vi "通道配置模块.vi"() -> (1 "返回":bool)   [LabVIEW 2010]
uses:
  全局量/试验配置信息.vi
  全局量/全局_配置.vi
  <vilib>/Utility/config.llb/Write Key (String).vi
  <vilib>/Utility/config.llb/Write Key (I32).vi
  <vilib>/Utility/config.llb/NI_LVConfig.lvlib
panel:
  out "temp":string[](array[string])
  in  "Row":i32
  in  "模拟量误差":dbl format="%.4f"
  out "配置文件目录":path
  out "配置文件路径":path
  out "配置文件目录 2":path
  out "配置文件路径 2":path
  in  "选项卡控件 2":enum32{"选项卡 1", "选项卡 2"}(tab)
  in  "模拟量误差百分比":dbl
  in  "数字量输出路数":u32=1 max=76
  in  "数字量输入路数":u32 max=80
  in  "DSP输入路数":u32 max=16
  in  "DSP输入幅值":enum32{"0-3V"}(ring)
  in  "AD输入路数":u32 max=16
  in  "AD输入幅值":enum32{"±3V", "±5V", "±12V"}(ring)
  in  "RS232路数":u32=1 max=2
  in  "RS485路数":u32=1 max=1
  in  "CAN路数":u32=1 max=4
  in  "btn_保存配置":bool
  in  "加载配置文件列表":u16(ring)
  in  "保存配置文件名称":string
  in  "选项卡控件":enum32{"测试类型Ⅰ", "测试类型Ⅱ", "测试类型Ⅲ", "测试类型Ⅳ"}(tab)
  in  "类型1测试路数":i32=1 min=0 max=16
  in  "D_IN_1":string[][](table) caption="表格"
  in  "类型2测试路数":i32=1 min=0 max=16
  in  "D_IN_2":string[][](table) caption="表格"
  in  "类型3测试路数":i32=1 min=0 max=80
  in  "D_IN_3":string[][](table) caption="表格"
  in  "类型4测试路数":i32=1 min=0 max=16
  in  "D_IN_4":string[][](table) caption="表格"
  in  "btn_保存配置 2":bool
  in  "加载配置文件列表 2":u16(ring)
  in  "保存配置文件名称 2":string
  in  "单选按钮":enum32{"单选选项1", "单选选项2"}(radio)
  in  "str_IP":string
  in  "单选_LAN":bool
  in  "CAN波特率":T1(ring)
  in  "LAN端口":u32
  in  "RS485_2端口":refnum<visa-resource-name>="COM1"
  in  "RS485_1端口":refnum<visa-resource-name>="COM1"
  in  "RS485波特率":T2(ring)
  in  "R232端口":refnum<visa-resource-name>="COM1"
  in  "btn_返回":bool
  # "板卡测试配置"
  # "控制板IP："
  # "控制板端口："
  # "COM端口："
  # "1号"
  # "COM端口："
  # "2号"
  # "CAN总线通信波特率："
  # "RS485总线通信波特率："
  # "数字量输出信号路数："
  # "数字量输入信号路数："
  # "外部AD模拟量输入信号路数："
  # "DSP模拟量输入信号路数："
  # "外部AD模拟量输入信号幅值："
  # "DSP模拟量输入信号幅值："
  # "RS232总线通信路数："
  # "RS485总线通信路数："
  # "CAN总线通信路数："
  # "模拟量允许误差："
  # "%"
  # "加载配置文件："
  # "保存配置文件名称："
  # "C1-"
  # "加载配置文件："
  # "保存配置文件名称："
  # "C2-"
  # "测试路数："
  # "测试类型I函数：y =f1(A1*x+A2)\ny:模拟量输入\nx:模拟量输出"
  # "测试路数："
  # "测试路数："
  # "测试类型III函数：y =f3(x)\ny:数字量输入\nx:数字量输出\n是否锁定=1，y=锁定值；\n是否锁定=0，mode=1，y=~x；\n是否锁定=0，mode=0，y=x；\n是否锁定=-1，mode=0，y=x；"
  # "测试路数："
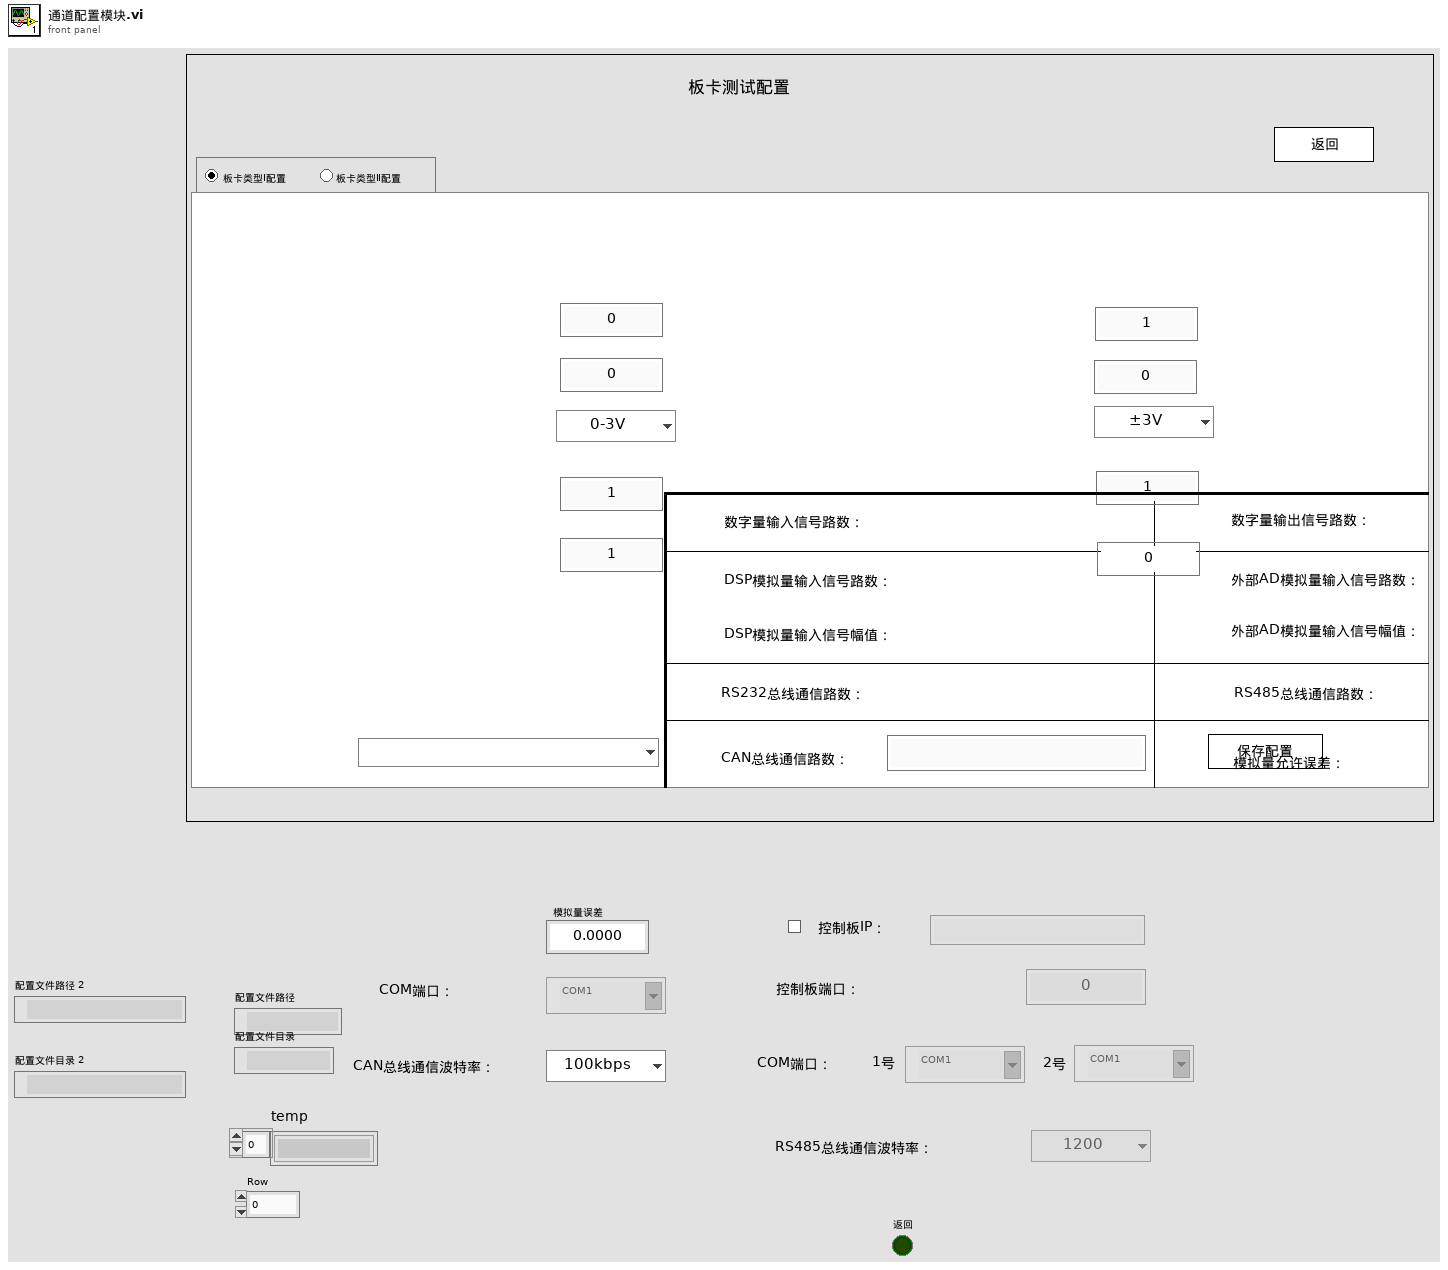
[diagram p1: front panel]
types:
  T1 = enum32{"100kbps", "200kbps", "250kbps", "500kbps", "1000kbps"}
  T2 = enum32{"1200", "2400", "4800", "9600", "19200", "57600", "115200", ""}
  T3 = enum8{"Enabled", "Disabled", "Disabled and Grayed Out"}
  T4 = cluster{"数字量输入信号路数":i32, "数字量输出信号路数":i32, "DSP模拟量输入信号路数":u32, "DSP模拟量输入信号幅值":u32, "AD模拟量输入信号路数":u32, "AD模拟量输入信号幅值":u32, "RS232端口":u32, "RS232通信路数":u32, "RS232波特率":dbl, "RS485端口":u32, "RS485通信路数":u32, "RS485波特率":u32, "CAN通信路数":i32, "CAN波特率":u32, "以太网选择?":bool, "控制板IP":string, "以太网端口":u32}
  T5 = cluster{"数字量输入路数":u32, "数字量输出路数":u32, "DSP输入路数":u32, "DSP输入幅值":enum32{"0-3V"}, "AD输入路数":u32, "AD输入幅值":enum32{"±3V", "±5V", "±12V"}, "毫秒倍数":u32, "RS232路数":u32, "模拟量误差":dbl, "毫秒倍数":u32, "RS485路数":u32, "RS485波特率":enum32{"1200", "2400", "4800", "9600", "19200", "57600", "115200", ""}, "CAN路数":u32, "CAN波特率":enum32{"100kbps", "200kbps", "250kbps", "500kbps", "1000kbps"}, "单选_LAN":bool, "str_IP":string, "LAN端口":u32}
  T6 = typedef "NI_LVConfig.lvlib/Config Data RefNum.ctl" = refnum<k1>
  T7 = typedef "LVPoint32TypeDef.ctl" = cluster{"Horizontal":i32, "Vertical":i32}
  T8 = typedef "LVRowAndColumnTypeDef.ctl" = cluster{"Row":i32, "Column":i32}
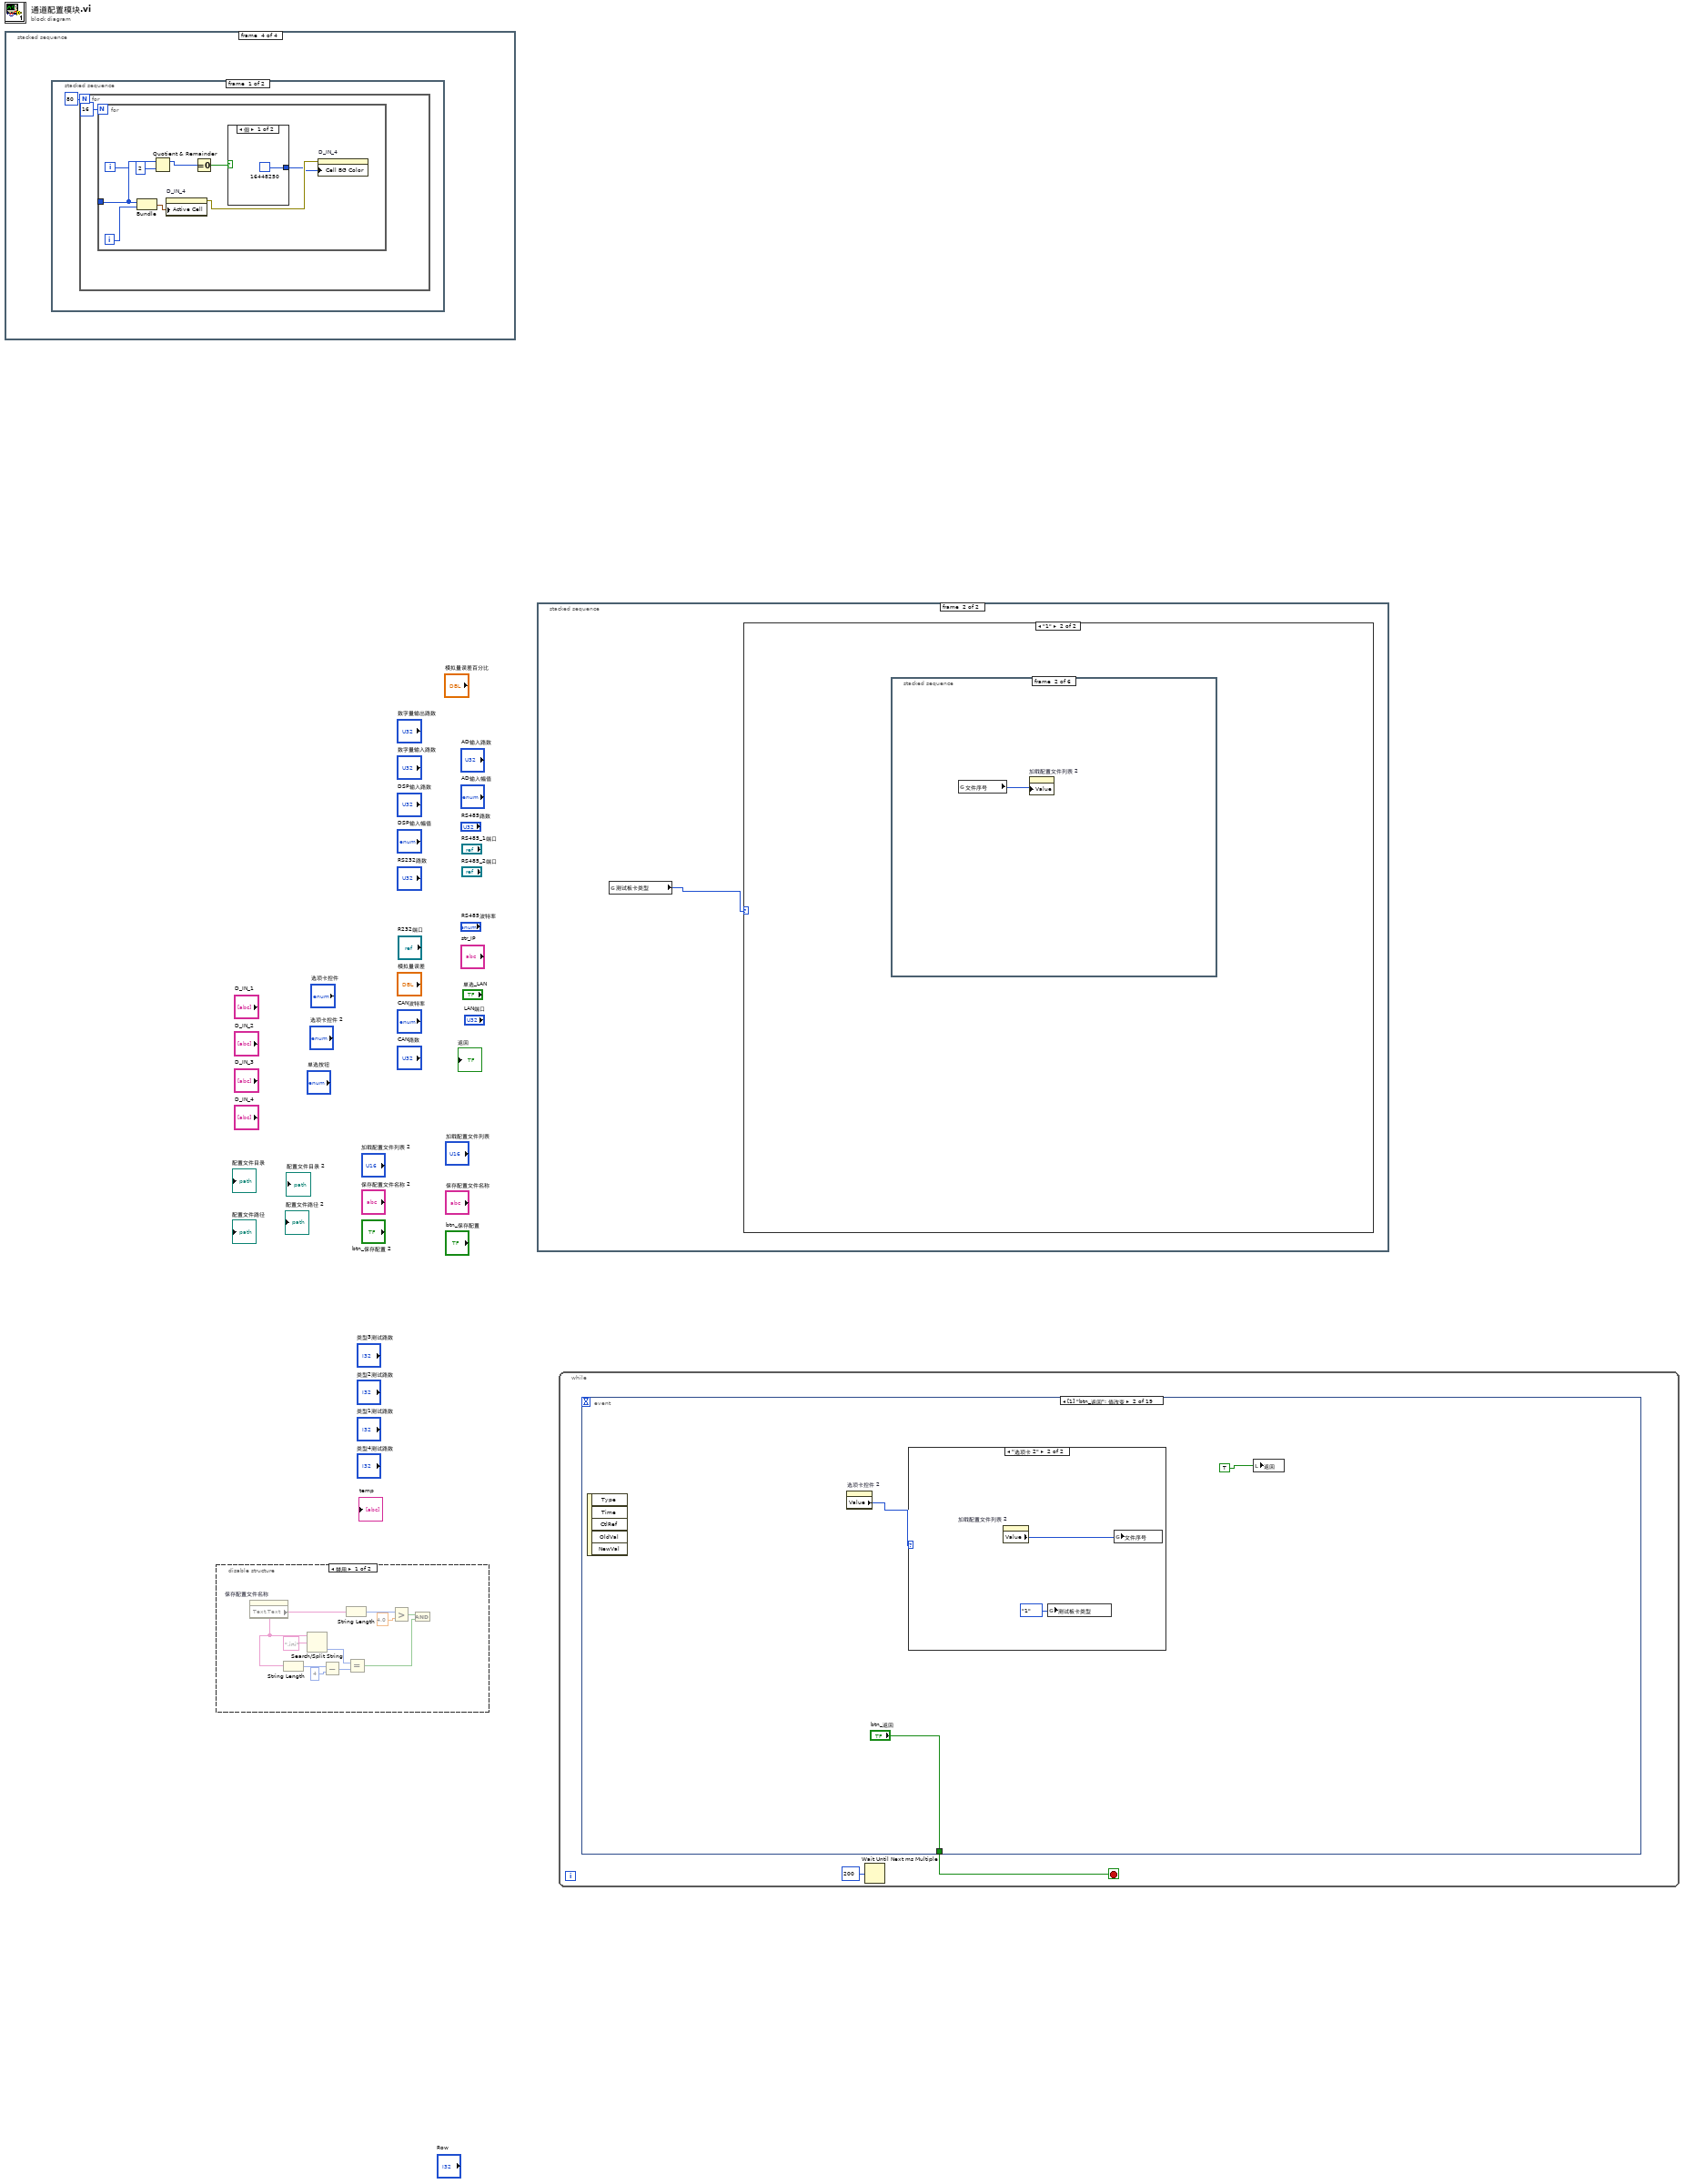
[diagram p0: block diagram]
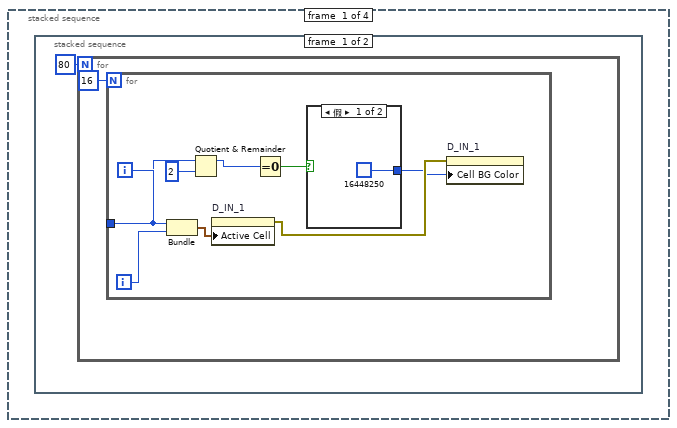
[diagram p2: hidden frame]
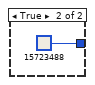
[diagram p3: hidden frame]
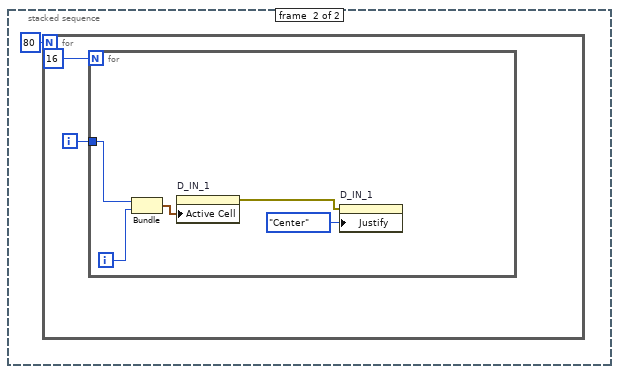
[diagram p4: hidden frame]
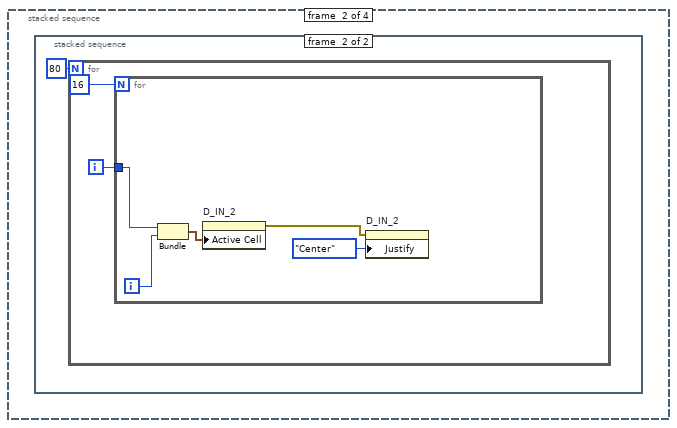
[diagram p5: hidden frame]
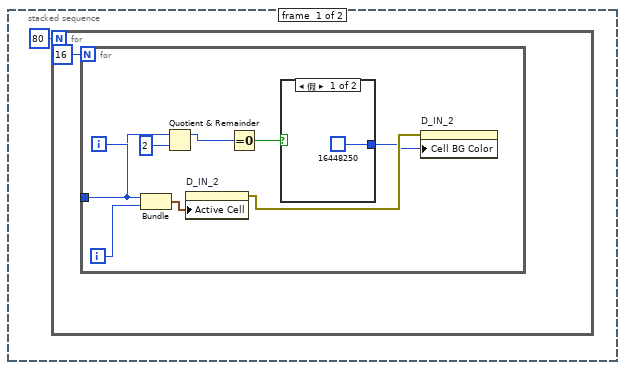
[diagram p6: hidden frame]
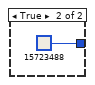
[diagram p7: hidden frame]
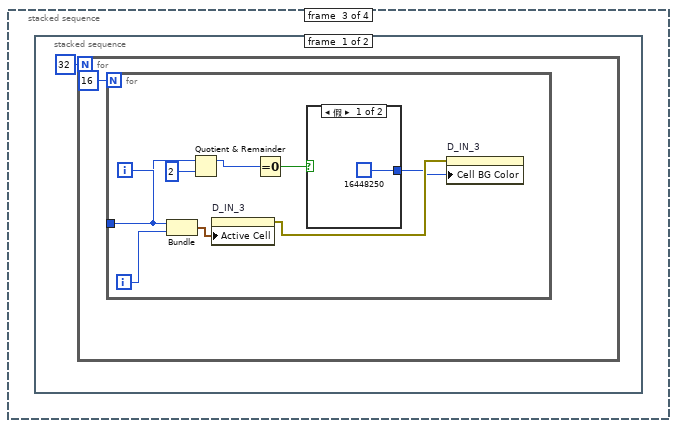
[diagram p8: hidden frame]
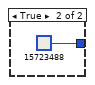
[diagram p9: hidden frame]
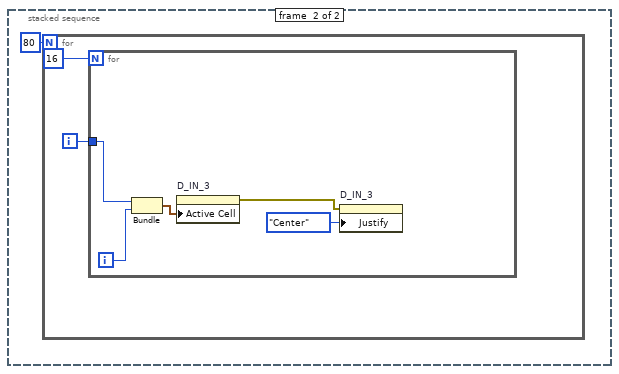
[diagram p10: hidden frame]
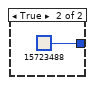
[diagram p11: hidden frame]
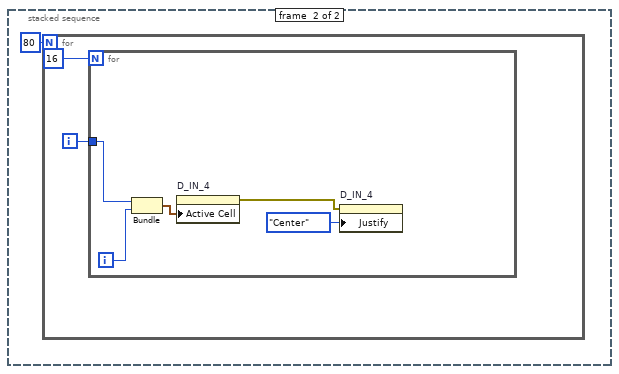
[diagram p12: hidden frame]
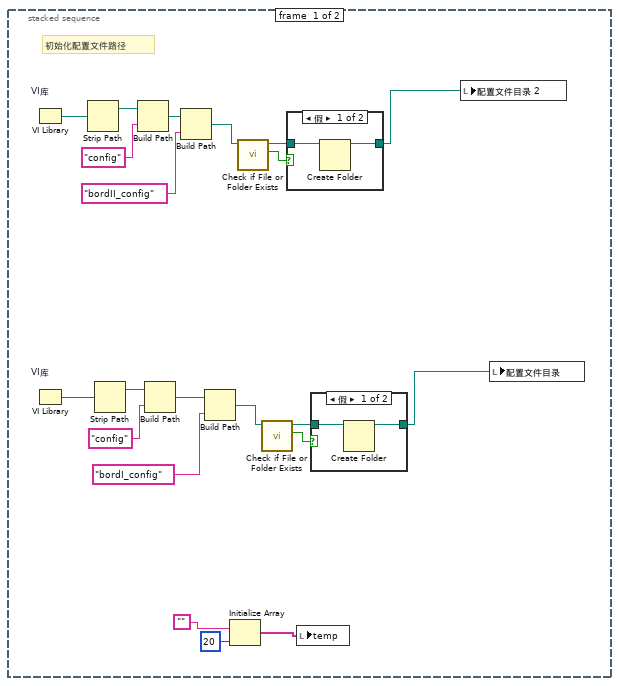
[diagram p14: hidden frame]
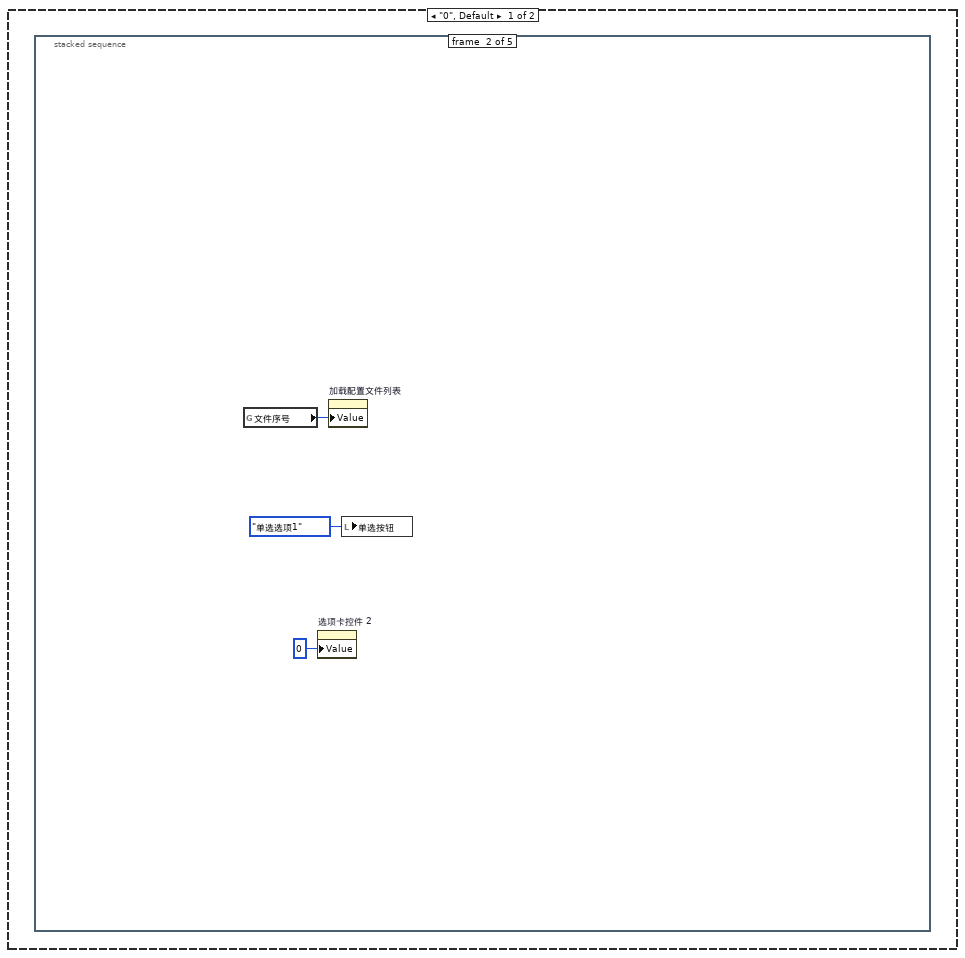
[diagram p17: hidden frame]
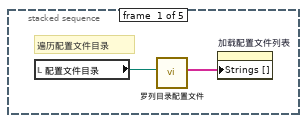
[diagram p18: hidden frame]
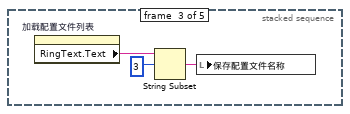
[diagram p19: hidden frame]
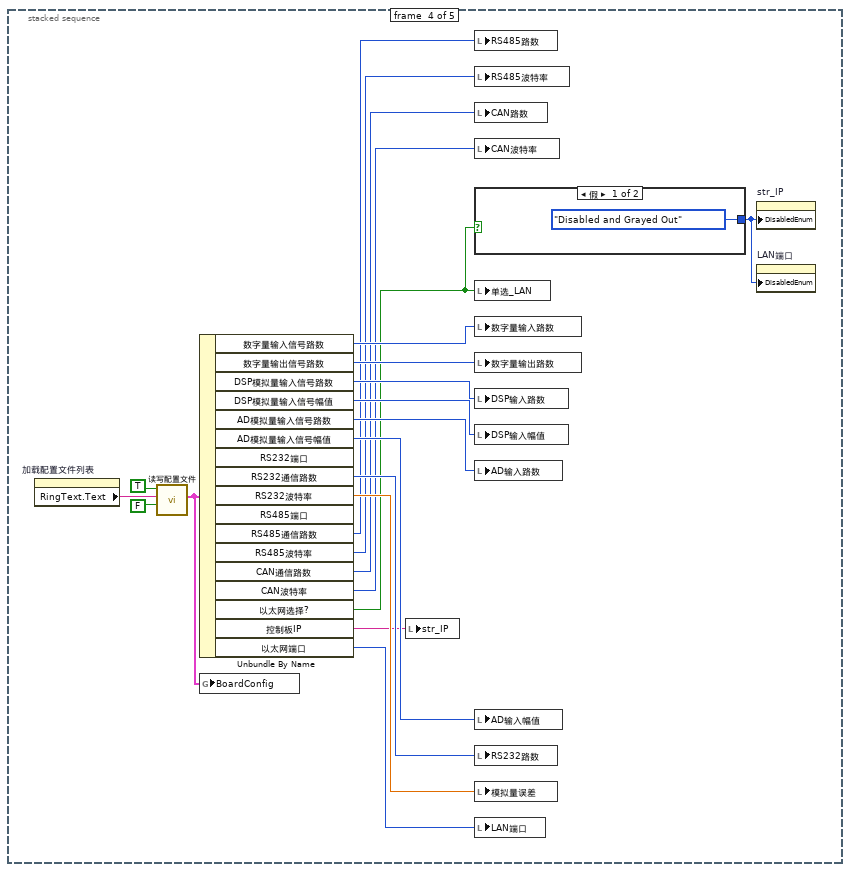
[diagram p20: hidden frame]
diagram:
  n1 = stacked-sequence {
    frame #0 {
      n2 = stacked-sequence {
        frame #0 {
          n3 = for {
            N: 80 -> [_]
            i -> [w3]
            n4 = for {
              N: 16 -> [_]
              tunnel: w3 -> [w10]
              i -> [w4]
              n5 = Bundle(w10, w4) -> (w7:cluster{i32, i32})  [unwired: 1 in]
              n6 = Quotient & Remainder(x=w10, y=2) -> (x-y*floor(x/y)=w8:i32)  [unwired: 1 out]
              n7 = property on="D_IN_1" class="Tbl (严格)"("Active Cell"=w7) -> (error out=w6:errorcluster)  [unwired: 2 in, 1 out]
              n8 = Equal To 0?(x=w8) -> (x = 0?=w11:bool)
              n9 = case shown="假" w11 {
                tunnel: [u32 16448250 u32 15723488] -> w5
                frame False {
                }
                frame True {
                }
              }
              n10 = property on="D_IN_1" class="Tbl (严格)"(error in=w6, "Cell BG Color"=w5) -> ()  [unwired: 1 in, 2 out]
            }
          }
        }
        frame #1 {
          n11 = for {
            N: 80 -> [_]
            i -> [w15]
            n12 = for {
              N: 16 -> [_]
              tunnel: w15 -> [w17]
              i -> [w18]
              n13 = Bundle(w17, w18) -> (w21:cluster{i32, i32})  [unwired: 1 in]
              n14 = property on="D_IN_1" class="Tbl (严格)"("Active Cell"=w21) -> (error out=w19:errorcluster)  [unwired: 2 in, 1 out]
              n15 = property on="D_IN_1" class="Tbl (严格)"(error in=w19, "Justify"=enum16{"Left", "Center", "Right"}."Center" ("活动单元格:单元格对齐")) -> ()  [unwired: 1 in, 2 out]
            }
          }
        }
      }
    }
    frame #1 {
      n16 = stacked-sequence {
        frame #0 {
          n17 = for {
            N: 80 -> [_]
            i -> [w24]
            n18 = for {
              N: 16 -> [_]
              tunnel: w24 -> [w31]
              i -> [w25]
              n19 = Bundle(w31, w25) -> (w28:cluster{i32, i32})  [unwired: 1 in]
              n20 = Quotient & Remainder(x=w31, y=2) -> (x-y*floor(x/y)=w29:i32)  [unwired: 1 out]
              n21 = property on="D_IN_2" class="Tbl (严格)"("Active Cell"=w28) -> (error out=w27:errorcluster)  [unwired: 2 in, 1 out]
              n22 = Equal To 0?(x=w29) -> (x = 0?=w32:bool)
              n23 = case shown="假" w32 {
                tunnel: [u32 16448250 u32 15723488] -> w26
                frame False {
                }
                frame True {
                }
              }
              n24 = property on="D_IN_2" class="Tbl (严格)"(error in=w27, "Cell BG Color"=w26) -> ()  [unwired: 1 in, 2 out]
            }
          }
        }
        frame #1 {
          n25 = for {
            N: 80 -> [_]
            i -> [w36]
            n26 = for {
              N: 16 -> [_]
              tunnel: w36 -> [w38]
              i -> [w39]
              n27 = Bundle(w38, w39) -> (w42:cluster{i32, i32})  [unwired: 1 in]
              n28 = property on="D_IN_2" class="Tbl (严格)"("Active Cell"=w42) -> (error out=w40:errorcluster)  [unwired: 2 in, 1 out]
              n29 = property on="D_IN_2" class="Tbl (严格)"(error in=w40, "Justify"=enum16{"Left", "Center", "Right"}."Center" ("活动单元格:单元格对齐")) -> ()  [unwired: 1 in, 2 out]
            }
          }
        }
      }
    }
    frame #2 {
      n30 = stacked-sequence {
        frame #0 {
          n31 = for {
            N: 32 -> [_]
            i -> [w45]
            n32 = for {
              N: 16 -> [_]
              tunnel: w45 -> [w52]
              i -> [w46]
              n33 = Bundle(w52, w46) -> (w49:cluster{i32, i32})  [unwired: 1 in]
              n34 = Quotient & Remainder(x=w52, y=2) -> (x-y*floor(x/y)=w50:i32)  [unwired: 1 out]
              n35 = property on="D_IN_3" class="Tbl (严格)"("Active Cell"=w49) -> (error out=w48:errorcluster)  [unwired: 2 in, 1 out]
              n36 = Equal To 0?(x=w50) -> (x = 0?=w53:bool)
              n37 = case shown="假" w53 {
                tunnel: [u32 16448250 u32 15723488] -> w47
                frame False {
                }
                frame True {
                }
              }
              n38 = property on="D_IN_3" class="Tbl (严格)"(error in=w48, "Cell BG Color"=w47) -> ()  [unwired: 1 in, 2 out]
            }
          }
        }
        frame #1 {
          n39 = for {
            N: 80 -> [_]
            i -> [w57]
            n40 = for {
              N: 16 -> [_]
              tunnel: w57 -> [w59]
              i -> [w60]
              n41 = Bundle(w59, w60) -> (w63:cluster{i32, i32})  [unwired: 1 in]
              n42 = property on="D_IN_3" class="Tbl (严格)"("Active Cell"=w63) -> (error out=w61:errorcluster)  [unwired: 2 in, 1 out]
              n43 = property on="D_IN_3" class="Tbl (严格)"(error in=w61, "Justify"=enum16{"Left", "Center", "Right"}."Center" ("活动单元格:单元格对齐")) -> ()  [unwired: 1 in, 2 out]
            }
          }
        }
      }
    }
    frame #3 {
      n44 = stacked-sequence {
        frame #0 {
          n45 = for {
            N: 80 -> [_]
            i -> [w66]
            n46 = for {
              N: 16 -> [_]
              tunnel: w66 -> [w73]
              i -> [w67]
              n47 = Bundle(w73, w67) -> (w70:cluster{i32, i32})  [unwired: 1 in]
              n48 = Quotient & Remainder(x=w73, y=2) -> (x-y*floor(x/y)=w71:i32)  [unwired: 1 out]
              n49 = property on="D_IN_4" class="Tbl (严格)"("Active Cell"=w70) -> (error out=w69:errorcluster)  [unwired: 2 in, 1 out]
              n50 = Equal To 0?(x=w71) -> (x = 0?=w74:bool)
              n51 = case shown="假" w74 {
                tunnel: [u32 16448250 u32 15723488] -> w68
                frame False {
                }
                frame True {
                }
              }
              n52 = property on="D_IN_4" class="Tbl (严格)"(error in=w69, "Cell BG Color"=w68) -> ()  [unwired: 1 in, 2 out]
            }
          }
        }
        frame #1 {
          n53 = for {
            N: 80 -> [_]
            i -> [w78]
            n54 = for {
              N: 16 -> [_]
              tunnel: w78 -> [w80]
              i -> [w81]
              n55 = Bundle(w80, w81) -> (w84:cluster{i32, i32})  [unwired: 1 in]
              n56 = property on="D_IN_4" class="Tbl (严格)"("Active Cell"=w84) -> (error out=w82:errorcluster)  [unwired: 2 in, 1 out]
              n57 = property on="D_IN_4" class="Tbl (严格)"(error in=w82, "Justify"=enum16{"Left", "Center", "Right"}."Center" ("活动单元格:单元格对齐")) -> ()  [unwired: 1 in, 2 out]
            }
          }
        }
      }
    }
  }
  n58 = disable-structure shown="禁用" {
    frame Disabled {
      n59 = property on="保存配置文件名称" class="Str"() -> ("Text.Text"=w90:string)  [unwired: 2 in, 2 out]
      n60 = String Length(string=w90) -> (length=w91:i32)
      n61 = Search/Split String(string=w90, search string/char (-)=".ini" ("搜索字符串/字符(-)")) -> (offset of match=w89:i32)  [unwired: 1 in, 2 out]
      n62 = Subtract(x=w91, y=4) -> (x-y=w93:i32)
      n63 = String Length(string=w90) -> (length=w87:i32)
      n64 = Equal?(x=w89, y=w93) -> (x = y?=w94:bool)
      n65 = Greater?(x=w87, y=4.0) -> (0:w88:bool)
      n66 = And(x=w88, y=w94) -> ()  [unwired: 1 out]
    }
    frame Enabled {
    }
  }
  n67 = stacked-sequence {
    frame #0 {
      # "初始化配置文件路径"
      n68 = VI Library "VI库"() -> (path=w103:path)
      n69 = VI Library "VI库"() -> (path=w115:path)
      n70 = Strip Path(path=w103) -> (stripped path=w102:path)  [unwired: 1 out]
      n71 = Strip Path(path=w115) -> (stripped path=w114:path)  [unwired: 1 out]
      n72 = Build Path(base path=w102, name or relative path="config" ("名称或相对路径")) -> (appended path=w100:path)
      n73 = Build Path(base path=w114, name or relative path="config" ("名称或相对路径")) -> (appended path=w107:path)
      n74 = Build Path(base path=w100, name or relative path="bordII_config" ("名称或相对路径")) -> (appended path=w96:path)
      n75 = Build Path(base path=w107, name or relative path="bordI_config" ("名称或相对路径")) -> (appended path=w109:path)
      n76 = Initialize Array("", 20 ("维数大小")) -> (w106:string[])
      n77 = call <vilib>:"Check if File or Folder Exists.vi"("path"=w96) -> ("file or folder exists?"=w97:bool, "dup path"=w98:path)  [unwired: 8 in, 1 out]
      n78 = call <vilib>:"Check if File or Folder Exists.vi"("path"=w109) -> ("file or folder exists?"=w110:bool, "dup path"=w111:path)  [unwired: 8 in, 1 out]
      n79 = case shown="假" w97 {
        tunnel: w98 -> [w116 w118]
        tunnel: [w117 w118] -> w95
        frame False {
          n80 = Create Folder(path (use dialog)=w116) -> (created path=w117:path)  [unwired: 2 in, 2 out]
        }
        frame True {
        }
      }
      n81 = local write "temp"(w106) -> ()
      n82 = case shown="假" w110 {
        tunnel: w111 -> [w119 w121]
        tunnel: [w120 w121] -> w108
        frame False {
          n83 = Create Folder(path (use dialog)=w119) -> (created path=w120:path)  [unwired: 2 in, 2 out]
        }
        frame True {
        }
      }
      n84 = local write "配置文件目录 2"(w95) -> ()
      n85 = local write "配置文件目录"(w108) -> ()
    }
    frame #1 {
      n86 = global read "试验配置信息.vi" "测试板卡类型"() -> (w122:enum16{"0", "1"})
      n87 = case shown="\"1\"" w122 {
        frame "0", Default {
          n88 = stacked-sequence {
            frame #0 {
              # "遍历配置文件目录"
              n89 = local read "配置文件目录"() -> (w124:path)
              n90 = call "罗列目录配置文件.vi"("路径"=w124) -> ("数组"=w123:string[])  [unwired: 10 in]
              n91 = property on="加载配置文件列表" class="Ring (严格)"("Strings []"=w123) -> ()  [unwired: 2 in, 2 out]
            }
            frame #1 {
              n92 = global read "试验配置信息.vi" "文件序号"() -> (w126:i32)
              n93 = property on="选项卡控件 2" class="TabCtl (严格)"("Value"=0) -> ()  [unwired: 2 in, 2 out]
              n94 = property on="加载配置文件列表" class="Ring (严格)"("Value"=w126) -> ()  [unwired: 2 in, 2 out]
              n95 = local write "单选按钮"(enum32{"单选选项1", "单选选项2"}."单选选项1" ("单选按钮")) -> ()
            }
            frame #2 {
              n96 = property on="加载配置文件列表" class="Ring (严格)"() -> ("RingText.Text"=w130:string)  [unwired: 2 in, 2 out]
              n97 = String Subset(string=w130, offset (0)=3 ("偏移量(0)")) -> (substring=w129:string)  [unwired: 1 in]
              n98 = local write "保存配置文件名称"(w129) -> ()
            }
            frame #3 {
              n99 = property on="加载配置文件列表" class="Ring (严格)"() -> ("RingText.Text"=w131:string)  [unwired: 2 in, 2 out]
              n100 = call "读写配置文件.vi"("m_bCreat"=FALSE ("m_bRead"), "文件名称"=w131, "m_bRead"=TRUE) -> ("BoardConfig_output"=w133:T4)  [unwired: 8 in]
              n101 = Unbundle By Name(w133) -> ("数字量输入信号路数"=w149:i32, "数字量输出信号路数"=w148:i32, "DSP模拟量输入信号路数"=w144:u32, "DSP模拟量输入信号幅值"=w147:u32, "AD模拟量输入信号路数"=w146:u32, "AD模拟量输入信号幅值"=w145:u32, "RS232通信路数"=w143:u32, "RS232波特率"=w142:dbl, "RS485通信路数"=w141:u32, "RS485波特率"=w140:u32, "CAN通信路数"=w139:i32, "CAN波特率"=w138:u32, "以太网选择?"=w135:bool, "控制板IP"=w137:string, "以太网端口"=w136:u32)  [unwired: 2 out]
              n102 = global write "全局_配置.vi" "BoardConfig"(w133) -> ()
              n103 = local write "str_IP"(w137) -> ()
              n104 = local write "RS485路数"(w141) -> ()
              n105 = local write "RS485波特率"(w140) -> ()
              n106 = local write "CAN路数"(w139) -> ()
              n107 = local write "CAN波特率"(w138) -> ()
              n108 = case shown="假" w135 {
                tunnel: [T3."Disabled and Grayed Out" ("禁用") T3."Enabled" ("禁用")] -> w134
                frame False {
                }
                frame True {
                }
              }
              n109 = local write "单选_LAN"(w135) -> ()
              n110 = local write "数字量输入路数"(w149) -> ()
              n111 = local write "数字量输出路数"(w148) -> ()
              n112 = local write "DSP输入路数"(w144) -> ()
              n113 = local write "DSP输入幅值"(w147) -> ()
              n114 = local write "AD输入路数"(w146) -> ()
              n115 = local write "AD输入幅值"(w145) -> ()
              n116 = local write "RS232路数"(w143) -> ()
              n117 = local write "模拟量误差"(w142) -> ()
              n118 = local write "LAN端口"(w136) -> ()
              n119 = property on="str_IP" class="Str"("DisabledEnum"=w134) -> ()  [unwired: 2 in, 2 out]
              n120 = property on="LAN端口" class="DigNum (严格)"("DisabledEnum"=w134) -> ()  [unwired: 2 in, 2 out]
            }
            frame #4 {
              n121 = local read "模拟量误差"() -> (w155:dbl)
              n122 = Multiply(x=w155, y=100.0) -> (x*y=w153:dbl)
              n123 = local write "模拟量误差百分比"(w153) -> ()
            }
          }
        }
        frame "1" {
          n124 = stacked-sequence {
            frame #0 {
              n125 = local write "单选按钮"(enum32{"单选选项1", "单选选项2"}."单选选项2" ("单选按钮")) -> ()
              n126 = property on="选项卡控件 2" class="TabCtl (严格)"("Value"=1) -> ()  [unwired: 2 in, 2 out]
            }
            frame #1 {
              n127 = global read "试验配置信息.vi" "文件序号"() -> (w158:i32)
              n128 = property on="加载配置文件列表 2" class="Ring (严格)"("Value"=w158) -> ()  [unwired: 2 in, 2 out]
            }
            frame #2 {
              # "遍历配置文件目录"
              n129 = local read "配置文件目录 2"() -> (w160:path)
              n130 = call "罗列目录配置文件.vi"("路径"=w160) -> ("数组"=w159:string[])  [unwired: 10 in]
              n131 = property on="加载配置文件列表 2" class="Ring (严格)"("Strings []"=w159) -> ()  [unwired: 2 in, 2 out]
            }
            frame #3 {
              n132 = property on="加载配置文件列表 2" class="Ring (严格)"() -> ("RingText.Text"=w162:string)  [unwired: 2 in, 2 out]
              n133 = String Subset(string=w162, offset (0)=3 ("偏移量(0)")) -> (substring=w163:string)  [unwired: 1 in]
              n134 = local write "保存配置文件名称 2"(w163) -> ()
            }
            frame #4 {
              # "待读取配置文件路径"
              n135 = local read "配置文件目录 2"() -> (w165:path)
              n136 = property on="加载配置文件列表 2" class="Ring (严格)"() -> ("RingText.Text"=w164:string)  [unwired: 2 in, 2 out]
              n137 = Build Path(base path=w165, name or relative path=w164) -> (appended path=w166:path)
              n138 = local write "配置文件路径 2"(w166) -> ()
            }
            frame #5 {
              # "读取默认配置的配置内容"
              n139 = local read "配置文件路径 2"() -> (w167:path)
              n140 = call "函数测试配置文件读取.vi"("配置文件路径"=w167) -> ("类型1路数"=w172:i32, "类型2路数"=w173:i32, "类型3路数"=w174:i32, "类型4路数"=w175:i32, "D_IN_1"=w168:string[][], "D_IN_2"=w169:string[][], "D_IN_3"=w170:string[][], "D_IN_4"=w171:string[][])  [unwired: 11 in]
              n141 = local write "D_IN_1"(w168) -> ()
              n142 = local write "D_IN_2"(w169) -> ()
              n143 = local write "D_IN_3"(w170) -> ()
              n144 = local write "D_IN_4"(w171) -> ()
              n145 = global write "试验配置信息.vi" "自测类型4路数"(w175) -> ()
              n146 = local write "类型4测试路数"(w175) -> ()
              n147 = global write "试验配置信息.vi" "自测类型3路数"(w174) -> ()
              n148 = local write "类型3测试路数"(w174) -> ()
              n149 = global write "试验配置信息.vi" "自测类型2路数"(w173) -> ()
              n150 = local write "类型2测试路数"(w173) -> ()
              n151 = global write "试验配置信息.vi" "自测类型1路数"(w172) -> ()
              n152 = local write "类型1测试路数"(w172) -> ()
            }
          }
        }
      }
    }
  }
  n153 = while {
    stop <- w177 stop-if-true
    n154 = event shown="[1] \"btn_返回\": 值改变" {
      selector: _ -> [_ _ _ _ _ _ _ _ _ _ _ _ _ _ _ _ _ _ _]
      dyn-events: _ -> [_ _ _ _ _ _ _ _ _ _ _ _ _ _ _ _ _ _ _]
      timeout: _ -> [_ _ _ _ _ _ _ _ _ _ _ _ _ _ _ _ _ _ _]
      tunnel: [_ "btn_返回" _ _ _ _ _ _ _ _ _ _ _ _ _ _ _ _ TRUE] -> w177
      event Timeout {
        n155 = event-data() -> ()  [unwired: 1 in, 2 out]
      }
      event "btn_返回": Value Change {
        n156 = event-data() -> ()  [unwired: 1 in, 5 out]
        n157 = property on="选项卡控件 2" class="TabCtl (严格)"() -> ("Value"=w179:enum32{"选项卡 1", "选项卡 2"})  [unwired: 2 in, 2 out]
        n158 = case shown="\"选项卡 2\"" w179 {
          frame "选项卡 1", Default {
            n159 = local read "加载配置文件列表"() -> (w182:u16)
            n160 = global write "试验配置信息.vi" "测试板卡类型"(enum16{"0", "1"}."0" ("测试板卡类型")) -> ()
            n161 = global write "试验配置信息.vi" "文件序号"(w182) -> ()
          }
          frame "选项卡 2" {
            n162 = property on="加载配置文件列表 2" class="Ring (严格)"() -> ("Value"=w183:u16)  [unwired: 2 in, 2 out]
            n163 = global write "试验配置信息.vi" "测试板卡类型"(enum16{"0", "1"}."1" ("测试板卡类型")) -> ()
            n164 = global write "试验配置信息.vi" "文件序号"(w183) -> ()
          }
        }
        n165 = local write "返回"(TRUE) -> ()
      }
      event "btn_保存配置": Mouse Up {
        n166 = event-data() -> ()  [unwired: 1 in, 7 out]
        n167 = call "显示对话框信息2"() -> ("确定"=w185:bool)  [unwired: 10 in, 1 out]
        n168 = case shown="真" w185 {
          frame False {
          }
          frame True {
            n169 = stacked-sequence {
              frame #0 {
                n170 = local read "模拟量误差百分比"() -> (w188:dbl)
                n171 = Divide(x=w188, y=100.0) -> (x/y=w186:dbl)
                n172 = local write "模拟量误差"(w186) -> ()
              }
              frame #1 {
                n173 = local read "数字量输入路数"() -> (w200:u32)
                n174 = local read "数字量输出路数"() -> (w199:u32)
                n175 = local read "RS485波特率"() -> (w212:T2)
                n176 = local read "DSP输入路数"() -> (w198:u32)
                n177 = local read "DSP输入幅值"() -> (w203:enum32{"0-3V"})
                n178 = local read "模拟量误差"() -> (w201:dbl)
                n179 = local read "AD输入路数"() -> (w197:u32)
                n180 = local read "AD输入幅值"() -> (w202:enum32{"±3V", "±5V", "±12V"})
                n181 = local read "CAN波特率"() -> (w211:T1)
                n182 = local read "RS232路数"() -> (w196:u32)
                n183 = local read "RS485路数"() -> (w195:u32)
                n184 = local read "单选_LAN"() -> (w210:bool)
                n185 = local read "CAN路数"() -> (w194:u32)
                n186 = local read "LAN端口"() -> (w208:u32)
                n187 = local read "str_IP"() -> (w209:string)
                n188 = Bundle("数字量输入路数"=w200, "数字量输出路数"=w199, "DSP输入路数"=w198, "DSP输入幅值"=w203, "AD输入路数"=w197, "AD输入幅值"=w202, "毫秒倍数"=u32 0, "RS232路数"=w196, "模拟量误差"=w201, "毫秒倍数"=u32 0, "RS485路数"=w195, "RS485波特率"=w212, "CAN路数"=w194, "CAN波特率"=w211, "单选_LAN"=w210, "str_IP"=w209, "LAN端口"=w208) -> (w206:T5)  [unwired: 1 in]
                n189 = global write "全局_配置.vi" "BoardConfig"(w206) -> ()
                n190 = case shown="\"0-3V\", 默认" w203 {
                  tunnel: [3.3] -> w204
                  frame "0-3V", Default {
                  }
                }
                n191 = case shown="\"±12V\"" w202 {
                  tunnel: [6.0 10.0 24.0] -> w205
                  frame "±3V", Default {
                  }
                  frame "±5V" {
                  }
                  frame "±12V" {
                  }
                }
                n192 = global write "全局_配置.vi" "ad模拟量输入路数"(w197) -> ()
                n193 = global write "全局_配置.vi" "模拟量误差"(w201) -> ()
                n194 = global write "全局_配置.vi" "R485路数"(w195) -> ()
                n195 = global write "试验配置信息.vi" "自测CAN路数"(w194) -> ()
                n196 = global write "全局_配置.vi" "数字量输入路数"(w200) -> ()
                n197 = global write "全局_配置.vi" "数字量输出路数"(w199) -> ()
                n198 = global write "全局_配置.vi" "dsp模拟量输入路数"(w198) -> ()
                n199 = global write "全局_配置.vi" "R232路数"(w196) -> ()
                n200 = global write "全局_配置.vi" "DSP模拟量量程范围"(w204) -> ()
                n201 = global write "全局_配置.vi" "ARM模拟量量程范围"(w205) -> ()
                n202 = local read "保存配置文件名称"() -> (w190:string)
                n203 = local write "返回"(TRUE) -> ()
                n204 = Concatenate Strings("C1-", w190) -> (w189:string)
                n205 = call "读写配置文件.vi"("BoardConfig_input"=w206, "m_bCreat"=TRUE, "文件名称"=w189, "m_bRead"=FALSE) -> ()  [unwired: 7 in, 1 out]
              }
              frame #2 {
                # "遍历配置文件目录"
                n206 = local read "配置文件目录"() -> (w219:path)
                n207 = call "罗列目录配置文件.vi"("路径"=w219) -> ("数组"=w220:string[])  [unwired: 10 in]
                n208 = property on="加载配置文件列表" class="Ring (严格)"("Strings []"=w220) -> ()  [unwired: 2 in, 2 out]
              }
              frame #3 {
                n209 = local read "加载配置文件列表"() -> (w222:u16)
                n210 = global write "试验配置信息.vi" "测试板卡类型"(enum16{"0", "1"}."0" ("测试板卡类型")) -> ()
                n211 = global write "试验配置信息.vi" "文件序号"(w222) -> ()
              }
            }
          }
        }
      }
      event "btn_保存配置 2": Mouse Up {
        n212 = event-data() -> ()  [unwired: 1 in, 7 out]
        n213 = call "显示对话框信息4"() -> ("确定"=w223:bool)  [unwired: 10 in, 1 out]
        n214 = case shown="真" w223 {
          frame False {
          }
          frame True {
            n215 = stacked-sequence {
              frame #0 {
                n216 = property on="保存配置文件名称 2" class="Str"() -> ("Text.Text"=w225:string)  [unwired: 2 in, 2 out]
                n217 = String Length(string=w225) -> (length=w226:i32)
                n218 = Greater?(x=w226, y=0.0) -> (0:w224:bool)
                n219 = case shown="真" w224 {
                  frame False {
                    n220 = call "显示对话框信息3"() -> ()  [unwired: 10 in, 2 out]
                  }
                  frame True {
                    n221 = stacked-sequence {
                      frame #0 {
                        # "待保存配置文件路径"
                        n222 = local read "保存配置文件名称 2"() -> (w229:string)
                        n223 = local read "配置文件目录 2"() -> (w232:path)
                        n224 = Concatenate Strings("C2-", w229) -> (w228:string)
                        n225 = Build Path(base path=w232, name or relative path=w228) -> (appended path=w231:path)
                        n226 = local write "配置文件路径 2"(w231) -> ()
                      }
                      frame #1 {
                        w233 = "TEST_CONFIG" ("section")
                        n227 = local read "配置文件路径 2"() -> (w276:path)
                        n228 = local read "D_IN_1"() -> (w273:string[][])
                        n229 = local read "D_IN_2"() -> (w264:string[][])
                        n230 = local read "D_IN_3"() -> (w258:string[][])
                        n231 = local read "D_IN_4"() -> (w252:string[][])
                        n232 = call <vilib>:"Open Config Data.vi"("configuration file path"=w276) -> ("error out"=w275:errorcluster, "refnum"=w274:T6)  [unwired: 8 in, 1 out]
                        n233 = Array To Spreadsheet String(array=w273, 3:"%s" ("格式字符串")) -> (spreadsheet string=w271:string)  [unwired: 1 in]
                        n234 = call-poly <vilib>:"Write Key.vi"("section"=w233, "error in (no error)"=w275, "value"=w271, "key"="test1", "refnum"=w274) -> ("error out"=w266:errorcluster, "refnum out"=w267:T6)  [unwired: 4 in, 1 out]
                        n235 = Array To Spreadsheet String(array=w264, 3:"%s" ("格式字符串")) -> (spreadsheet string=w268:string)  [unwired: 1 in]
                        n236 = call-poly <vilib>:"Write Key.vi"("section"=w233, "error in (no error)"=w266, "value"=w268, "key"="test2", "refnum"=w267) -> ("error out"=w259:errorcluster, "refnum out"=w260:T6)  [unwired: 4 in, 1 out]
                        n237 = Array To Spreadsheet String(array=w258, 3:"%s" ("格式字符串")) -> (spreadsheet string=w262:string)  [unwired: 1 in]
                        n238 = call-poly <vilib>:"Write Key.vi"("section"=w233, "error in (no error)"=w259, "value"=w262, "key"="test3", "refnum"=w260) -> ("error out"=w253:errorcluster, "refnum out"=w254:T6)  [unwired: 4 in, 1 out]
                        n239 = Array To Spreadsheet String(array=w252, 3:"%s" ("格式字符串")) -> (spreadsheet string=w256:string)  [unwired: 1 in]
                        n240 = call-poly <vilib>:"Write Key.vi"("section"=w233, "error in (no error)"=w253, "value"=w256, "key"="test4", "refnum"=w254) -> ("error out"=w250:errorcluster, "refnum out"=w251:T6)  [unwired: 4 in, 1 out]
                        n241 = local read "类型3测试路数"() -> (w240:i32)
                        n242 = local read "类型4测试路数"() -> (w236:i32)
                        n243 = local read "类型1测试路数"() -> (w249:i32)
                        n244 = call-poly <vilib>:"Write Key.vi"("section"=w233, "error in (no error)"=w250, "value"=w249, "key"="test1_num", "refnum"=w251) -> ("error out"=w247:errorcluster, "refnum out"=w246:T6)  [unwired: 4 in, 1 out]
                        n245 = local read "类型2测试路数"() -> (w244:i32)
                        n246 = call-poly <vilib>:"Write Key.vi"("section"=w233, "error in (no error)"=w247, "value"=w244, "key"="test2_num", "refnum"=w246) -> ("error out"=w242:errorcluster, "refnum out"=w243:T6)  [unwired: 4 in, 1 out]
                        n247 = call-poly <vilib>:"Write Key.vi"("section"=w233, "error in (no error)"=w242, "value"=w240, "key"="test3_num", "refnum"=w243) -> ("error out"=w238:errorcluster, "refnum out"=w239:T6)  [unwired: 4 in, 1 out]
                        n248 = call-poly <vilib>:"Write Key.vi"("section"=w233, "error in (no error)"=w238, "value"=w236, "key"="test4_num", "refnum"=w239) -> ("error out"=w235:errorcluster, "refnum out"=w234:T6)  [unwired: 4 in, 1 out]
                        n249 = call <vilib>:"Close Config Data.vi"("error in (no error)"=w235, "refnum"=w234) -> ()  [unwired: 8 in, 2 out]
                        n250 = global write "试验配置信息.vi" "自测类型1路数"(w249) -> ()
                        n251 = global write "试验配置信息.vi" "自测类型2路数"(w244) -> ()
                        n252 = global write "试验配置信息.vi" "自测类型3路数"(w240) -> ()
                        n253 = global write "试验配置信息.vi" "自测类型4路数"(w236) -> ()
                      }
                      frame #2 {
                        # "刷新下拉列表"
                        n254 = local read "配置文件目录 2"() -> (w278:path)
                        n255 = call "罗列目录配置文件.vi"("路径"=w278) -> ("数组"=w277:string[])  [unwired: 10 in]
                        n256 = property on="加载配置文件列表 2" class="Ring (严格)"("Strings []"=w277) -> ()  [unwired: 2 in, 2 out]
                      }
                      frame #3 {
                        # "选中当前配置文件"
                        n257 = property on="保存配置文件名称 2" class="Str"() -> ("Text.Text"=w279:string)  [unwired: 2 in, 2 out]
                        n258 = property on="加载配置文件列表 2" class="Ring (严格)"("RingText.Text"=w279) -> ()  [unwired: 2 in, 2 out]
                      }
                      frame #4 {
                        n259 = local read "配置文件目录"() -> (w285:path)
                        n260 = call "罗列目录配置文件.vi"("路径"=w285) -> ("数组"=w284:string[])  [unwired: 10 in]
                        n261 = global write "试验配置信息.vi" "测试板卡类型"(enum16{"0", "1"}."1" ("测试板卡类型")) -> ()
                        n262 = property on="加载配置文件列表 2" class="Ring (严格)"() -> ("Value"=w282:u16)  [unwired: 2 in, 2 out]
                        n263 = Array Size(array=w284) -> (size(s)=w283:i32)
                        n264 = Add(x=w282, y=w283) -> (x+y=w281:i32)
                        n265 = global write "试验配置信息.vi" "文件序号"(w281) -> ()
                      }
                      frame #5 {
                        n266 = local read "D_IN_1"() -> (w290:string[][])
                        n267 = local read "D_IN_2"() -> (w289:string[][])
                        n268 = local read "D_IN_3"() -> (w288:string[][])
                        n269 = local read "D_IN_4"() -> (w287:string[][])
                        n270 = global write "试验配置信息.vi" "D_IN_1"(w290) -> ()
                        n271 = global write "试验配置信息.vi" "D_IN_2"(w289) -> ()
                        n272 = global write "试验配置信息.vi" "D_IN_3"(w288) -> ()
                        n273 = global write "试验配置信息.vi" "D_IN_4"(w287) -> ()
                        n274 = local write "返回"(TRUE) -> ()
                      }
                    }
                  }
                }
              }
            }
          }
        }
      }
      event "单选_LAN": Value Change {
        n275 = event-data() -> ("NewVal"=w291:bool)  [unwired: 1 in, 4 out]
        n276 = case shown="假" w291 {
          tunnel: [T3."Disabled and Grayed Out" ("禁用") T3."Enabled" ("禁用")] -> w292
          frame False {
          }
          frame True {
          }
        }
        n277 = property on="str_IP" class="Str"("DisabledEnum"=w292) -> ()  [unwired: 2 in, 2 out]
        n278 = property on="LAN端口" class="DigNum (严格)"("DisabledEnum"=w292) -> ()  [unwired: 2 in, 2 out]
      }
      event "RS485路数": Value Change {
        n279 = event-data() -> ()  [unwired: 1 in, 5 out]
        n280 = disable-structure shown="禁用" {
          frame Disabled {
            n281 = case shown="\"1\"" {
              selector: _ -> [_ _]
              tunnel: [w297 T3."Disabled" ("禁用")] -> w296
              tunnel: [w297 T3."Disabled" ("禁用")] -> w295
              tunnel: [w297 T3."Disabled and Grayed Out" ("禁用")] -> _
              frame "1", Default {
                w297 = T3."Disabled and Grayed Out" ("禁用")
              }
              frame "1" {
              }
            }
            n282 = property on="RS485波特率" class="Enum (严格)"("DisabledEnum"=w295) -> ()  [unwired: 2 in, 2 out]
            n283 = property on="RS485_1端口" class="VISAName"("DisabledEnum"=w296) -> ()  [unwired: 2 in, 2 out]
          }
          frame Enabled {
          }
        }
      }
      event "RS232路数": Value Change {
        n284 = event-data() -> ()  [unwired: 1 in, 5 out]
        n285 = disable-structure shown="禁用" {
          frame Disabled {
            n286 = case shown="\"1\"" {
              selector: _ -> [_ _]
              tunnel: [T3."Disabled and Grayed Out" ("禁用") T3."Enabled" ("禁用")] -> w301
              frame "1", Default {
              }
              frame "1" {
              }
            }
            n287 = property on="R232端口" class="VISAName"("DisabledEnum"=w301) -> ()  [unwired: 2 in, 2 out]
          }
          frame Enabled {
          }
        }
      }
      event "加载配置文件列表": Value Change {
        n288 = event-data() -> ()  [unwired: 1 in, 5 out]
        n289 = stacked-sequence {
          frame #0 {
            n290 = property on="加载配置文件列表" class="Ring (严格)"() -> ("RingText.Text"=w305:string)  [unwired: 2 in, 2 out]
            n291 = property on="加载配置文件列表" class="Ring (严格)"() -> ("Value"=w307:u16)  [unwired: 2 in, 2 out]
            n292 = String Subset(string=w305, offset (0)=3 ("偏移量(0)")) -> (substring=w304:string)  [unwired: 1 in]
            n293 = local write "保存配置文件名称"(w304) -> ()
            n294 = global write "试验配置信息.vi" "文件序号"(w307) -> ()
          }
          frame #1 {
            n295 = property on="加载配置文件列表" class="Ring (严格)"() -> ("RingText.Text"=w308:string)  [unwired: 2 in, 2 out]
            n296 = call "读写配置文件.vi"("m_bCreat"=FALSE, "文件名称"=w308, "m_bRead"=TRUE) -> ("BoardConfig_output"=w310:T4)  [unwired: 8 in]
            n297 = global write "全局_配置.vi" "BoardConfig"(w310) -> ()
            n298 = Unbundle By Name(w310) -> ("数字量输入信号路数"=w311:i32, "数字量输出信号路数"=w312:i32, "DSP模拟量输入信号路数"=w316:u32, "DSP模拟量输入信号幅值"=w313:u32, "AD模拟量输入信号路数"=w314:u32, "AD模拟量输入信号幅值"=w315:u32, "RS232通信路数"=w317:u32, "RS232波特率"=w318:dbl, "RS485通信路数"=w319:u32, "RS485波特率"=w320:u32, "CAN通信路数"=w321:i32, "CAN波特率"=w322:u32, "以太网选择?"=w325:bool, "控制板IP"=w323:string, "以太网端口"=w324:u32)  [unwired: 2 out]
            n299 = local write "数字量输入路数"(w311) -> ()
            n300 = local write "数字量输出路数"(w312) -> ()
            n301 = local write "DSP输入路数"(w316) -> ()
            n302 = local write "DSP输入幅值"(w313) -> ()
            n303 = local write "AD输入路数"(w314) -> ()
            n304 = local write "AD输入幅值"(w315) -> ()
            n305 = local write "RS485波特率"(w320) -> ()
            n306 = local write "RS232路数"(w317) -> ()
            n307 = local write "模拟量误差"(w318) -> ()
            n308 = local write "CAN波特率"(w322) -> ()
            n309 = local write "RS485路数"(w319) -> ()
            n310 = local write "CAN路数"(w321) -> ()
            n311 = local write "单选_LAN"(w325) -> ()
            n312 = local write "LAN端口"(w324) -> ()
            n313 = local write "str_IP"(w323) -> ()
            n314 = case shown="假" w325 {
              tunnel: [T3."Disabled and Grayed Out" ("禁用") T3."Enabled" ("禁用")] -> w326
              frame False {
              }
              frame True {
              }
            }
            n315 = property on="str_IP" class="Str"("DisabledEnum"=w326) -> ()  [unwired: 2 in, 2 out]
            n316 = property on="LAN端口" class="DigNum (严格)"("DisabledEnum"=w326) -> ()  [unwired: 2 in, 2 out]
          }
          frame #2 {
            n317 = local read "模拟量误差"() -> (w333:dbl)
            n318 = Multiply(x=w333, y=100.0) -> (x*y=w331:dbl)
            n319 = global write "试验配置信息.vi" "测试板卡类型"(enum16{"0", "1"}."0" ("测试板卡类型")) -> ()
            n320 = local write "模拟量误差百分比"(w331) -> ()
          }
        }
      }
      event "加载配置文件列表 2": Value Change {
        n321 = event-data() -> ()  [unwired: 1 in, 5 out]
        n322 = stacked-sequence {
          frame #0 {
            n323 = local read "配置文件目录"() -> (w342:path)
            n324 = call "罗列目录配置文件.vi"("路径"=w342) -> ("数组"=w341:string[])  [unwired: 10 in]
            n325 = property on="加载配置文件列表 2" class="Ring (严格)"() -> ("Value"=w339:u16)  [unwired: 2 in, 2 out]
            n326 = Array Size(array=w341) -> (size(s)=w340:i32)
            n327 = Add(x=w339, y=w340) -> (x+y=w338:i32)
            n328 = property on="加载配置文件列表 2" class="Ring (严格)"() -> ("RingText.Text"=w335:string)  [unwired: 2 in, 2 out]
            n329 = global write "试验配置信息.vi" "文件序号"(w338) -> ()
            n330 = String Subset(string=w335, offset (0)=3 ("偏移量(0)")) -> (substring=w334:string)  [unwired: 1 in]
            n331 = local write "保存配置文件名称 2"(w334) -> ()
            n332 = global write "试验配置信息.vi" "测试板卡类型"(enum16{"0", "1"}."1" ("测试板卡类型")) -> ()
          }
          frame #1 {
            n333 = property on="加载配置文件列表 2" class="Ring (严格)"() -> ("RingText.Text"=w343:string)  [unwired: 2 in, 2 out]
            n334 = local read "配置文件目录 2"() -> (w345:path)
            n335 = Build Path(base path=w345, name or relative path=w343) -> (appended path=w344:path)
            n336 = local write "配置文件路径 2"(w344) -> ()
          }
          frame #2 {
            n337 = local read "配置文件路径 2"() -> (w346:path)
            n338 = call "函数测试配置文件读取.vi"("配置文件路径"=w346) -> ("类型1路数"=w351:i32, "类型2路数"=w352:i32, "类型3路数"=w353:i32, "类型4路数"=w354:i32, "D_IN_1"=w347:string[][], "D_IN_2"=w348:string[][], "D_IN_3"=w349:string[][], "D_IN_4"=w350:string[][])  [unwired: 11 in]
            n339 = local write "类型3测试路数"(w353) -> ()
            n340 = local write "D_IN_1"(w347) -> ()
            n341 = local write "D_IN_2"(w348) -> ()
            n342 = local write "D_IN_3"(w349) -> ()
            n343 = local write "D_IN_4"(w350) -> ()
            n344 = global write "试验配置信息.vi" "自测类型4路数"(w354) -> ()
            n345 = local write "类型4测试路数"(w354) -> ()
            n346 = global write "试验配置信息.vi" "自测类型3路数"(w353) -> ()
            n347 = global write "试验配置信息.vi" "自测类型2路数"(w352) -> ()
            n348 = local write "类型2测试路数"(w352) -> ()
            n349 = global write "试验配置信息.vi" "自测类型1路数"(w351) -> ()
            n350 = local write "类型1测试路数"(w351) -> ()
          }
        }
      }
      event "D_IN_1": Shortcut Menu Activation? {
        n351 = event-data() -> ("Coords"=w359:T7)  [unwired: 1 in, 5 out]
        n352 = invoke on="D_IN_1" class="Tbl (严格)" method="Point To Row Column"("Point"=w359) -> ("CellPosition"=w356:T8)  [unwired: 5 in, 5 out]
        n353 = Unbundle(w356) -> ("Row"=w358:i32)  [unwired: 1 out]
        n354 = Equal?(x=w358, y=-1) -> (x = y?=w355:bool)
        n355 = local write "Row"(w358) -> ()
        n356 = event-data("Discard?"=w355) -> ()  [unwired: 1 in, 1 out]
      }
      event "D_IN_2": Shortcut Menu Activation? {
        n357 = event-data() -> ("Coords"=w364:T7)  [unwired: 1 in, 5 out]
        n358 = invoke on="D_IN_2" class="Tbl (严格)" method="Point To Row Column"("Point"=w364) -> ("CellPosition"=w361:T8)  [unwired: 5 in, 5 out]
        n359 = Unbundle(w361) -> ("Row"=w363:i32)  [unwired: 1 out]
        n360 = Equal?(x=w363, y=-1) -> (x = y?=w360:bool)
        n361 = local write "Row"(w363) -> ()
        n362 = event-data("Discard?"=w360) -> ()  [unwired: 1 in, 1 out]
      }
      event "D_IN_3": Shortcut Menu Activation? {
        n363 = event-data() -> ("Coords"=w369:T7)  [unwired: 1 in, 5 out]
        n364 = invoke on="D_IN_3" class="Tbl (严格)" method="Point To Row Column"("Point"=w369) -> ("CellPosition"=w366:T8)  [unwired: 5 in, 5 out]
        n365 = Unbundle(w366) -> ("Row"=w368:i32)  [unwired: 1 out]
        n366 = Equal?(x=w368, y=-1) -> (x = y?=w365:bool)
        n367 = local write "Row"(w368) -> ()
        n368 = event-data("Discard?"=w365) -> ()  [unwired: 1 in, 1 out]
      }
      event "D_IN_4": Shortcut Menu Activation? {
        n369 = event-data() -> ("Coords"=w374:T7)  [unwired: 1 in, 5 out]
        n370 = invoke on="D_IN_4" class="Tbl (严格)" method="Point To Row Column"("Point"=w374) -> ("CellPosition"=w371:T8)  [unwired: 5 in, 5 out]
        n371 = Unbundle(w371) -> ("Row"=w373:i32)  [unwired: 1 out]
        n372 = Equal?(x=w373, y=-1) -> (x = y?=w370:bool)
        n373 = local write "Row"(w373) -> ()
        n374 = event-data("Discard?"=w370) -> ()  [unwired: 1 in, 1 out]
      }
      event "D_IN_1": Shortcut Menu Selection (User) {
        n375 = event-data() -> ("ItemTag"=w375:string)  [unwired: 1 in, 6 out]
        n376 = case shown="\"粘贴\"" w375 {
          frame "删除", Default {
            n377 = local read "D_IN_1"() -> (w377:string[][])
            n378 = local read "Row"() -> (w378:i32)
            n379 = Delete From Array(array=w377, index (row)=w378) -> (array with subset deleted=w376:string[][])  [unwired: 2 in, 1 out]
            n380 = local write "D_IN_1"(w376) -> ()
          }
          frame "复制" {
            n381 = local read "D_IN_1"() -> (w381:string[][])
            n382 = local read "Row"() -> (w380:i32)
            n383 = Index Array(array=w381, index (row)=w380) -> (element=w379:string[])  [unwired: 1 in]
            n384 = local write "temp"(w379) -> ()
          }
          frame "粘贴" {
            n385 = local read "D_IN_1"() -> (w382:string[][])
            n386 = local read "temp"() -> (w385:string[])
            n387 = local read "Row"() -> (w383:i32)
            n388 = Insert Into Array(array=w382, index (row)=w383, new element=w385) -> (w384:string[][])  [unwired: 1 in]
            n389 = local write "D_IN_1"(w384) -> ()
          }
        }
      }
      event "D_IN_2": Shortcut Menu Selection (User) {
        n390 = event-data() -> ("ItemTag"=w386:string)  [unwired: 1 in, 6 out]
        n391 = case shown="\"粘贴\"" w386 {
          frame "删除", Default {
            n392 = local read "D_IN_2"() -> (w388:string[][])
            n393 = local read "Row"() -> (w389:i32)
            n394 = Delete From Array(array=w388, index (row)=w389) -> (array with subset deleted=w387:string[][])  [unwired: 2 in, 1 out]
            n395 = local write "D_IN_2"(w387) -> ()
          }
          frame "复制" {
            n396 = local read "D_IN_2"() -> (w392:string[][])
            n397 = local read "Row"() -> (w391:i32)
            n398 = Index Array(array=w392, index (row)=w391) -> (element=w390:string[])  [unwired: 1 in]
            n399 = local write "temp"(w390) -> ()
          }
          frame "粘贴" {
            n400 = local read "D_IN_2"() -> (w393:string[][])
            n401 = local read "temp"() -> (w396:string[])
            n402 = local read "Row"() -> (w394:i32)
            n403 = Insert Into Array(array=w393, index (row)=w394, new element=w396) -> (w395:string[][])  [unwired: 1 in]
            n404 = local write "D_IN_2"(w395) -> ()
          }
        }
      }
      event "D_IN_3": Shortcut Menu Selection (User) {
        n405 = event-data() -> ("ItemTag"=w397:string)  [unwired: 1 in, 6 out]
        n406 = case shown="\"删除\", 默认" w397 {
          frame "删除", Default {
            n407 = local read "D_IN_3"() -> (w399:string[][])
            n408 = local read "Row"() -> (w400:i32)
            n409 = Delete From Array(array=w399, index (row)=w400) -> (array with subset deleted=w398:string[][])  [unwired: 2 in, 1 out]
            n410 = local write "D_IN_3"(w398) -> ()
          }
          frame "复制" {
            n411 = local read "D_IN_3"() -> (w403:string[][])
            n412 = local read "Row"() -> (w402:i32)
            n413 = Index Array(array=w403, index (row)=w402) -> (element=w401:string[])  [unwired: 1 in]
            n414 = local write "temp"(w401) -> ()
          }
          frame "粘贴" {
            n415 = local read "D_IN_3"() -> (w404:string[][])
            n416 = local read "temp"() -> (w407:string[])
            n417 = local read "Row"() -> (w405:i32)
            n418 = Insert Into Array(array=w404, index (row)=w405, new element=w407) -> (w406:string[][])  [unwired: 1 in]
            n419 = local write "D_IN_3"(w406) -> ()
          }
        }
      }
      event "D_IN_4": Shortcut Menu Selection (User) {
        n420 = event-data() -> ("ItemTag"=w408:string)  [unwired: 1 in, 6 out]
        n421 = case shown="\"删除\", 默认" w408 {
          frame "删除", Default {
            n422 = local read "D_IN_4"() -> (w410:string[][])
            n423 = local read "Row"() -> (w411:i32)
            n424 = Delete From Array(array=w410, index (row)=w411) -> (array with subset deleted=w409:string[][])  [unwired: 2 in, 1 out]
            n425 = local write "D_IN_4"(w409) -> ()
          }
          frame "复制" {
            n426 = local read "D_IN_4"() -> (w414:string[][])
            n427 = local read "Row"() -> (w413:i32)
            n428 = Index Array(array=w414, index (row)=w413) -> (element=w412:string[])  [unwired: 1 in]
            n429 = local write "temp"(w412) -> ()
          }
          frame "粘贴" {
            n430 = local read "D_IN_4"() -> (w415:string[][])
            n431 = local read "temp"() -> (w418:string[])
            n432 = local read "Row"() -> (w416:i32)
            n433 = Insert Into Array(array=w415, index (row)=w416, new element=w418) -> (w417:string[][])  [unwired: 1 in]
            n434 = local write "D_IN_4"(w417) -> ()
          }
        }
      }
      event "单选按钮": Value Change {
        n435 = event-data() -> ("NewVal"=w419:enum32{"单选选项1", "单选选项2"})  [unwired: 1 in, 4 out]
        n436 = case shown="\"单选选项2\"" w419 {
          frame "单选选项1", Default {
            n437 = local write "选项卡控件 2"(enum32{"选项卡 1", "选项卡 2"}."选项卡 1" ("选项卡控件 2")) -> ()
          }
          frame "单选选项2" {
            n438 = stacked-sequence {
              frame #0 {
                n439 = local write "选项卡控件 2"(enum32{"选项卡 1", "选项卡 2"}."选项卡 2" ("选项卡控件 2")) -> ()
              }
              frame #1 {
                n440 = stacked-sequence {
                  frame #0 {
                    # "遍历配置文件目录"
                    n441 = local read "配置文件目录 2"() -> (w422:path)
                    n442 = call "罗列目录配置文件.vi"("路径"=w422) -> ("数组"=w423:string[])  [unwired: 10 in]
                    n443 = property on="加载配置文件列表 2" class="Ring (严格)"("Strings []"=w423) -> ()  [unwired: 2 in, 2 out]
                  }
                  frame #1 {
                    n444 = stacked-sequence {
                      frame #0 {
                        # "初始化默认读取配置文件名称"
                        n445 = local write "加载配置文件列表 2"(0) -> ()
                      }
                      frame #1 {
                        n446 = property on="加载配置文件列表 2" class="Ring (严格)"() -> ("RingText.Text"=w426:string)  [unwired: 2 in, 2 out]
                        n447 = String Subset(string=w426, offset (0)=3 ("偏移量(0)")) -> (substring=w425:string)  [unwired: 1 in]
                        n448 = local write "保存配置文件名称 2"(w425) -> ()
                      }
                    }
                  }
                  frame #2 {
                    # "待读取配置文件路径"
                    n449 = property on="加载配置文件列表 2" class="Ring (严格)"() -> ("RingText.Text"=w428:string)  [unwired: 2 in, 2 out]
                    n450 = local read "配置文件目录 2"() -> (w429:path)
                    n451 = Build Path(base path=w429, name or relative path=w428) -> (appended path=w430:path)
                    n452 = local write "配置文件路径 2"(w430) -> ()
                  }
                  frame #3 {
                    # "读取默认配置的配置内容"
                    n453 = local read "配置文件路径 2"() -> (w431:path)
                    n454 = call "函数测试配置文件读取.vi"("配置文件路径"=w431) -> ("类型1路数"=w436:i32, "类型2路数"=w437:i32, "类型3路数"=w438:i32, "类型4路数"=w439:i32, "D_IN_1"=w432:string[][], "D_IN_2"=w433:string[][], "D_IN_3"=w434:string[][], "D_IN_4"=w435:string[][])  [unwired: 11 in]
                    n455 = local write "D_IN_1"(w432) -> ()
                    n456 = local write "D_IN_2"(w433) -> ()
                    n457 = local write "D_IN_3"(w434) -> ()
                    n458 = local write "D_IN_4"(w435) -> ()
                    n459 = local write "类型3测试路数"(w438) -> ()
                    n460 = global write "试验配置信息.vi" "自测类型4路数"(w439) -> ()
                    n461 = local write "类型4测试路数"(w439) -> ()
                    n462 = global write "试验配置信息.vi" "自测类型3路数"(w438) -> ()
                    n463 = global write "试验配置信息.vi" "自测类型2路数"(w437) -> ()
                    n464 = local write "类型2测试路数"(w437) -> ()
                    n465 = global write "试验配置信息.vi" "自测类型1路数"(w436) -> ()
                    n466 = local write "类型1测试路数"(w436) -> ()
                  }
                }
              }
            }
          }
        }
      }
      event Panel Close {
        n467 = event-data() -> ()  [unwired: 1 in, 3 out]
      }
    }
    n468 = Wait Until Next ms Multiple(millisecond multiple=u32 200 ("毫秒倍数")) -> ()  [unwired: 1 out]
  }
